vi "status scratch.vi"() -> ()   [LabVIEW 2011]
uses:
  DepthSense Global Status.vi
panel:
  out "Image":T1(plugin-control)
  in  "Image Height":i32
  in  "Image Width":i32
  in  "Minimum Framerate":i32
  in  "Maximum Framerate":i32
  in  "Framerate":i32=25
  in  "Close Mode":bool
  in  "Denoising":bool
  in  "Leakage Algorithm":bool
  in  "Anti-Aliasing":bool
  in  "Camera Status":i32
  in  "Camera Version":string
  in  "Light Intensity":i32=100
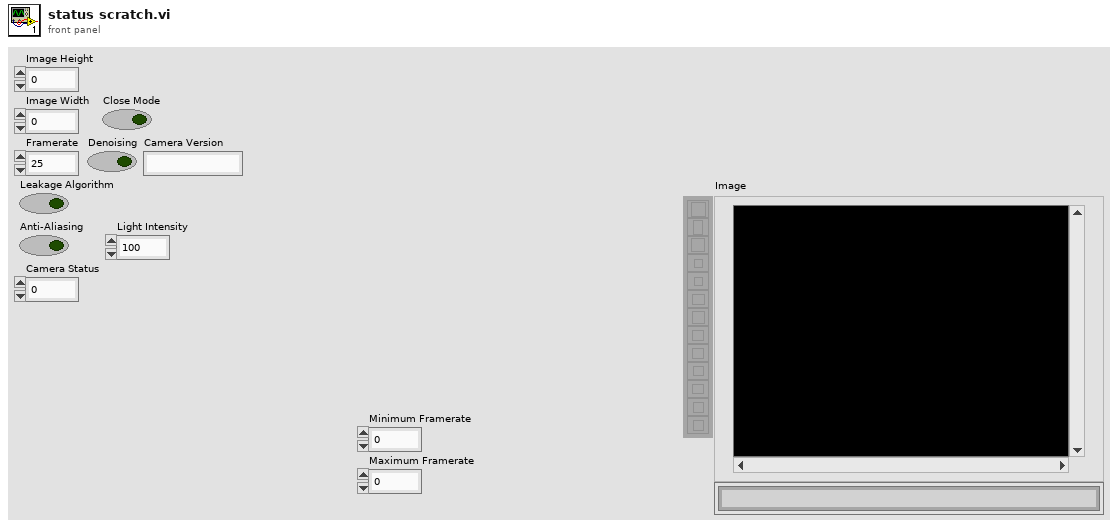
[diagram p1: front panel]
types:
  T1 = typedef "IMAQ Image.ctl" = refnum<image>
  T2 = typedef "Image Type" = u32
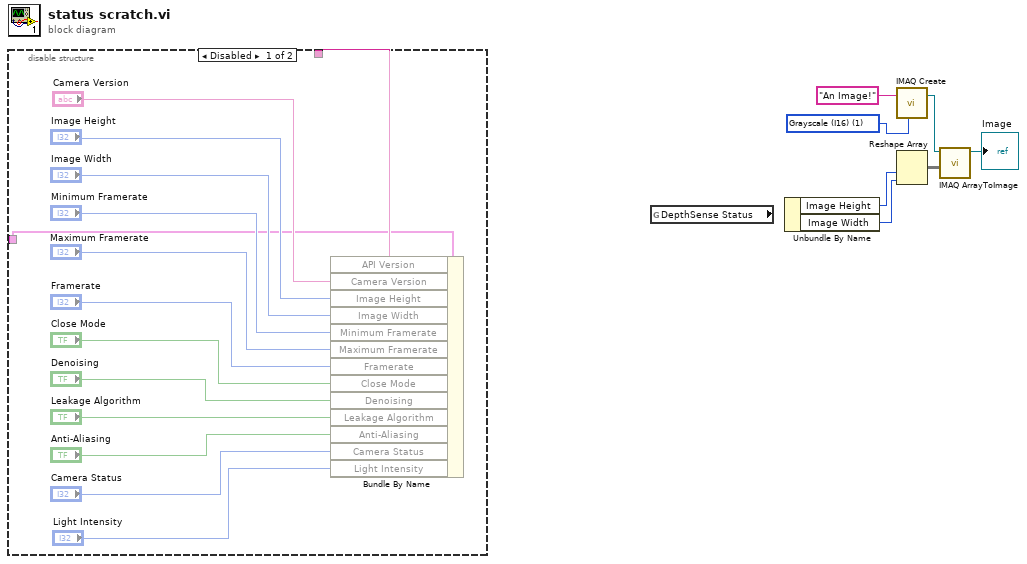
[diagram p0: block diagram]
diagram:
  w7 = T2 1 items=["Grayscale (U8)", "Grayscale (I16)", "Grayscale (SGL)", "Complex (CSG)", "RGB (U32)", "HSL (U32)", "RGB (U64)", "Grayscale (U16)"] ("Image Type")
  n1 = disable-structure shown="Disabled" {
    disable-tunnel: _ -> [w21 _]
    disable-tunnel: _ -> [w9 _]
    frame Disabled {
      n2 = Bundle By Name(cluster=w9, "API Version"=w21, "Camera Version"="Camera Version", "Image Height"="Image Height", "Image Width"="Image Width", "Minimum Framerate"="Minimum Framerate", "Maximum Framerate"="Maximum Framerate", "Framerate"="Framerate", "Close Mode"="Close Mode", "Denoising"="Denoising", "Leakage Algorithm"="Leakage Algorithm", "Anti-Aliasing"="Anti-Aliasing", "Camera Status"="Camera Status", "Light Intensity"="Light Intensity") -> ()  [unwired: 1 out]
    }
    frame Enabled {
    }
  }
  n3 = global read "DepthSense Global Status.vi" "DepthSense Status"() -> ()  [unwired: 1 out]
  n4 = Unbundle By Name() -> ("Image Height"=w2:i32, "Image Width"=w1:i32)  [unwired: 1 in]
  n5 = call "IMAQ Create"("Image Name"="An Image!", "Image Type"=w7) -> ("New Image"=w8:T1)  [unwired: 3 in, 1 out]
  n6 = Reshape Array(w2, w1) -> (w3:u16[], w5:void[][])
  n7 = call "IMAQ ArrayToImage"("Image Pixels (I16)"=w5, "Image"=w8) -> ("Image Out"=→"Image":T1)  [unwired: 8 in, 1 out]
